vi "Var_Axis.vi"(10 "Right Axis":u16[](array[numeric]), 11 "Left Axis":u16[](array[numeric])) -> (2 "Concatenate: Left = 0, Right = 1":i32[](array[numeric]), 3 "Concatenate":i32[](array[numeric]))   [LabVIEW 2019, in "Database Viewer.lvclass"]
uses:
  Database Viewer.lvclass
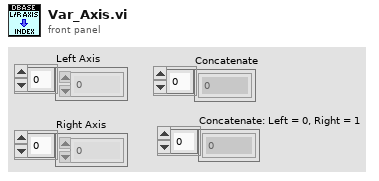
[diagram p1: front panel]
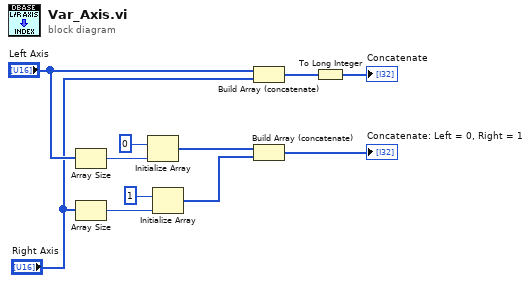
[diagram p0: block diagram]
diagram:
  n1 = Array Size(array="Left Axis") -> (size(s)=w6:i32)
  n2 = Array Size(array="Right Axis") -> (size(s)=w5:i32)
  n3 = Initialize Array(0 ("index"), w6) -> (w3:i32[])
  n4 = Initialize Array(1 ("index"), w5) -> (w4:i32[])
  n5 = Build Array (concatenate)("Left Axis", "Right Axis") -> (w10:u16[])
  n6 = Build Array (concatenate)(w3, w4) -> (→"Concatenate: Left = 0, Right = 1":i32[])
  n7 = To Long Integer(number=w10) -> (32bit integer=→"Concatenate":i32[])
